vi "RobotPositionReplacement.vi"(5 "How far behind":dbl=300.0 format="%#_13g", 7 "id":i32, 8 "IA State Input":T1, 9 "Position Ball":dbl[](array[numeric])) -> (2 "Position Robot":dbl[](array[numeric]))   [LabVIEW 2017]
uses:
  SSLView -Leonardo(GrSimTests)/Core/AI Input.ctl
  SSLView -Leonardo(GrSimTests)/Core/AI Robot.ctl
  SSLView -Leonardo(GrSimTests)/Intel/Functions Enum.ctl
  SSLView -Leonardo(GrSimTests)/Intel/AttackerStates.ctl
  SSLView -Leonardo(GrSimTests)/Path Planning/RRT/PathDests.ctl
  SSLView -Leonardo(GrSimTests)/Path Planning/RRT/PathDest.ctl
  SSLView -Leonardo(GrSimTests)/Core/AI Ball.ctl
  SSLView -Leonardo(GrSimTests)/Core/Field Size.ctl
  SSLView -Leonardo(GrSimTests)/Core/AI Judge.ctl
  SSLView -Leonardo(GrSimTests)/Intel/Command Enum.ctl
  SSLView -Leonardo(GrSimTests)/Util/Events/Events.ctl
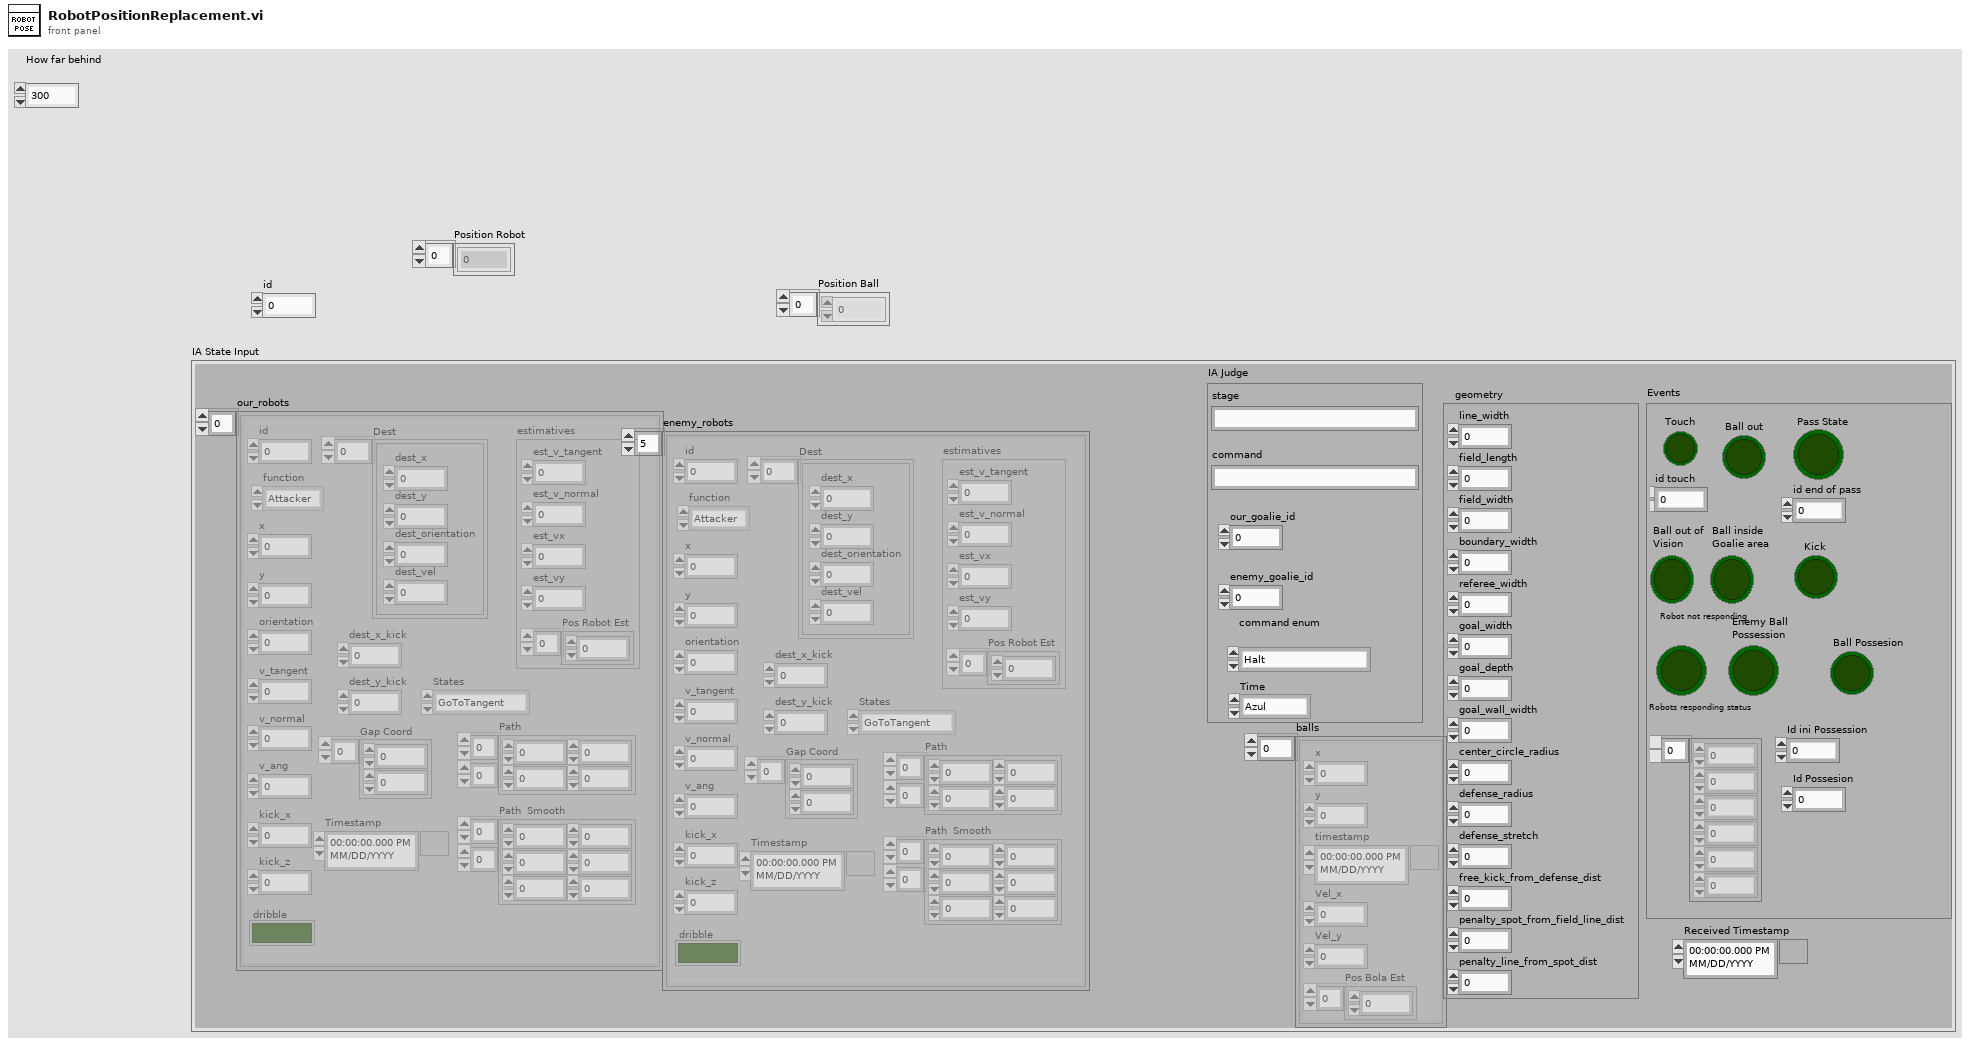
[diagram p1: front panel]
types:
  T1 = typedef "AI Input.ctl" = cluster{"our_robots":T2[], "enemy_robots":T2[], "balls":T7[], "geometry":T8, "IA Judge":T9, "Received Timestamp":timestamp, "Events":T11}
  T2 = typedef "AI Robot.ctl" = cluster{"id":u32, "function":T3, "x":dbl, "y":dbl, "orientation":dbl, "v_tangent":dbl, "v_normal":dbl, "v_ang":dbl, "kick_x":dbl, "kick_z":dbl, "dribble":bool, "Timestamp":timestamp, "estimatives":cluster{"est_v_tangent":dbl, "est_v_normal":dbl, "est_vx":dbl, "est_vy":dbl, "Pos Robot Est":dbl[]}, "dest_x_kick":dbl, "dest_y_kick":dbl, "Gap Coord":dbl[], "States":T4, "Path ":dbl[][], "Path  Smooth":dbl[][], "Dest":T5}
  T3 = typedef "Functions Enum.ctl" = enum16{"Attacker", "Goalie", "Defender", "Striker", "Goto 0", "Dummy", "Kicker", "ZigZag"}
  T4 = typedef "AttackerStates.ctl" = enum16{"Pass", "GoToTangent", "BallGetting", "GoToKick", ""}
  T5 = typedef "PathDests.ctl" = T6[]
  T6 = typedef "PathDest.ctl" = cluster{"dest_x":dbl, "dest_y":dbl, "dest_orientation":dbl, "dest_vel":dbl}
  T7 = typedef "AI Ball.ctl" = cluster{"x":dbl, "y":dbl, "timestamp":timestamp, "Vel_x":dbl, "Vel_y":dbl, "Pos Bola Est":dbl[]}
  T8 = typedef "Field Size.ctl" = cluster{"line_width":u32, "field_length":u32, "field_width":u32, "boundary_width":u32, "referee_width":u32, "goal_width":u32, "goal_depth":u32, "goal_wall_width":u32, "center_circle_radius":u32, "defense_radius":u32, "defense_stretch":u32, "free_kick_from_defense_dist":u32, "penalty_spot_from_field_line_dist":u32, "penalty_line_from_spot_dist":u32}
  T9 = typedef "AI Judge.ctl" = cluster{"stage":string, "command":string, "our_goalie_id":dbl, "enemy_goalie_id":dbl, "command enum":T10, "Time":enum16{"Azul", "Amarelo"}}
  T10 = typedef "Command Enum.ctl" = enum16{"Halt", "Stop", "Force Start", "PKA Normal Start", "Prepare Kickoff Ally", "PKE Normal Start", "Prepare Kickoff Enemy", "Prepare Penalty Ally", "PPA Normal Start", "Prepare Penalty Enemy", "PPE Normal Start", "Direct Free Enemy", "Direct Free Ally", "Indirect Free Enemy", "Indirect Free Ally", "Timeout Enemy", "Timeout Ally", "Goal Enemy", "Goal Ally", "Ball Placement Enemy", "Ball Placement Ally", "Normal Half Time", "Extra Time Break", "Extra Half Time", "None", "Post Game"}
  T11 = typedef "Events.ctl" = cluster{"Touch":bool, "Ball out":bool, "id touch":dbl, "Ball out of \nVision":bool, "Ball inside \nGoalie area":bool, "Robot not responding":bool, "Robots responding status":dbl[], "Enemy Ball \nPossession":bool, "Pass State":bool, "id end of pass":dbl, "Kick":bool, "Id ini Possession":dbl, "Ball Possesion":bool, "Id Possesion":dbl}
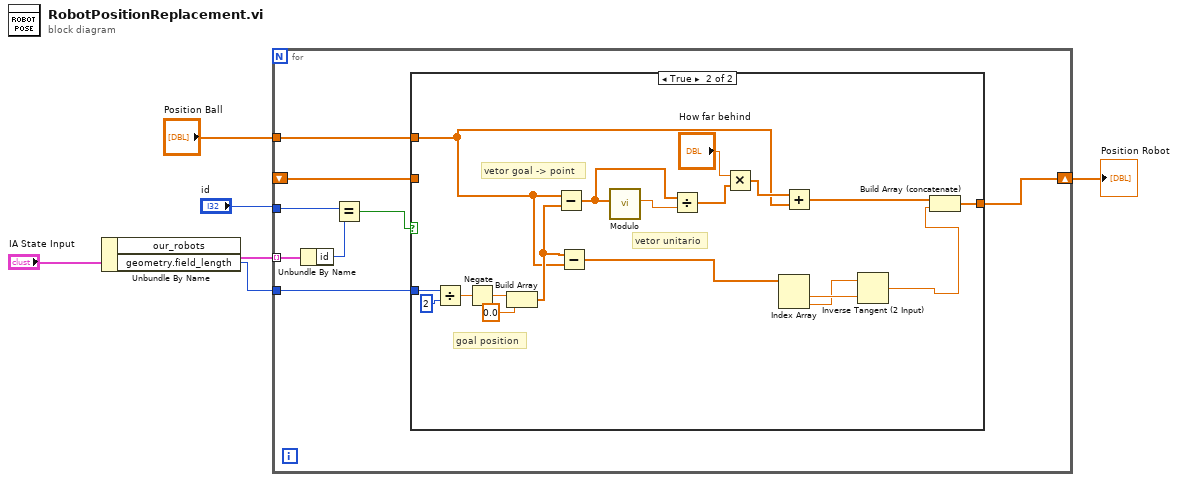
[diagram p0: block diagram]
diagram:
  n1 = Unbundle By Name("IA State Input") -> ("our_robots"=w5:T2[], "geometry.field_length"=w2:u32)
  n2 = for {
    tunnel: w5 -> [w11] mode=indexing
    tunnel: "id" -> [w14]
    tunnel: "Position Ball" -> [w12]
    tunnel: w2 -> [w9]
    shift-right: [w8] -> w1
    shift-left: _ -> [w7]
    n3 = Unbundle By Name(w11) -> ("id"=w10:u32)
    n4 = Equal?(x=w14, y=w10) -> (x = y?=w13:bool)
    n5 = case shown="True" w13 {
      tunnel: w12 -> [_ w18]
      tunnel: w9 -> [_ w33]
      tunnel: [w15 w23] -> w8
      tunnel: w7 -> [w15 _]
      frame False {
      }
      frame True {
        # "vetor unitario"
        # "vetor goal -> point"
        # "goal position"
        n6 = Divide(x=w33, y=u32 2) -> (x/y=w31:dbl)
        n7 = Negate(x=w31) -> (-x=w30:dbl)
        n8 = Build Array(w30, 0.0 ("element")) -> (w19:dbl[])
        n9 = Subtract(x=w18, y=w19) -> (x-y=w28:dbl[])
        n10 = Subtract(x=w19, y=w18) -> (x-y=w16:dbl[])
        n11 = call "Modulo.vi"("2D vector"=w28) -> ("Modulo"=w27:dbl)  [unwired: 10 in]
        n12 = Divide(x=w28, y=w27) -> (x/y=w17:dbl[])
        n13 = Multiply(x="How far behind", y=w17) -> (x*y=w25:dbl[])
        n14 = Index Array(array=w16) -> (element #1=w22:dbl, element #2=w21:dbl)  [unwired: 2 in]
        n15 = Add(x=w25, y=w18) -> (x+y=w24:dbl[])
        n16 = Inverse Tangent (2 Input)(1:w22, 2:w21) -> (0:w20:dbl)
        n17 = Build Array (concatenate)(w24, w20) -> (w23:dbl[])
      }
    }
  }
  "Position Robot" <- w1
